vi "QMH_releaseAll.vi"(8 "error in (no error)":errorcluster) -> (0 "error out":errorcluster)   [LabVIEW 2021, in "Framework_lib.lvlib"]
uses:
  Framework_lib.lvlib
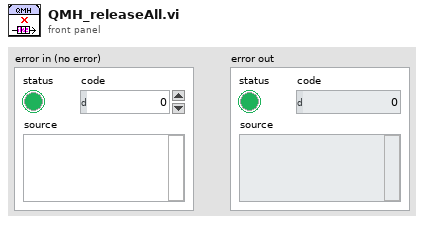
[diagram p1: front panel]
types:
  T1 = typedef "Framework_lib.lvlib/QMH_references.ctl" = cluster{"Consumer_SUT":refnum<queue>, "Consumer_annotation":refnum<queue>, "compute_results":refnum<queue>, "Notifier":refnum<notifier>}
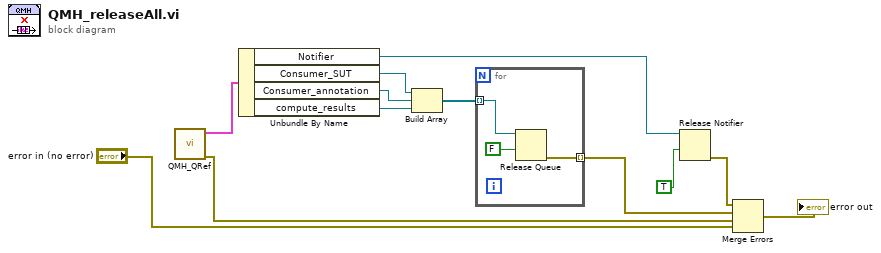
[diagram p0: block diagram]
diagram:
  n1 = call "QMH_QRef.vi"() -> ("error out"=w2:errorcluster, "Cluster Out"=w11:T1)  [unwired: 9 in, 1 out]
  n2 = Unbundle By Name(w11) -> ("Notifier"=w6:refnum<notifier>, "Consumer_SUT"=w10:refnum<queue>, "Consumer_annotation"=w9:refnum<queue>, "compute_results"=w8:refnum<queue>)
  n3 = Build Array(w10, w9, w8) -> (w7:refnum<queue>[])
  n4 = for {
    tunnel: w7 -> [w13] mode=indexing
    tunnel: [w15] -> w12 mode=indexing
    n5 = Release Queue(queue=w13, force destroy? (F)=FALSE) -> (error out=w15:errorcluster)  [unwired: 1 in, 2 out]
  }
  n6 = Release Notifier(notifier=w6, force destroy? (F)=TRUE) -> (error out=w4:errorcluster)  [unwired: 1 in, 2 out]
  n7 = Merge Errors(w4, w12, w2, "error in (no error)") -> (→"error out":errorcluster)
